vi "OE1022D_Common_Query Data.vi"(0 "VISA resource name":refnum<visa-resource-name>, 1 "OE1022D_Query Multi Data":T2 {"Query Type 5" items=["X", "Y", "R", "θ", "Freq", "Xh1", "Yh1", "Rh1", "θh1", "Xh2", "Yh2", "Rh2", "θh2", "Noise", "A1", "A2", "A3", "A4", "E1", "E2", "E3", "E4"]; "Query Type 4" items=["X", "Y", "R", "θ", "Freq", "Xh1", "Yh1", "Rh1", "θh1", "Xh2", "Yh2", "Rh2", "θh2", "Noise", "A1", "A2", "A3", "A4", "E1", "E2", "E3", "E4"]; "Query Type 3" items=["X", "Y", "R", "θ", "Freq", "Xh1", "Yh1", "Rh1", "θh1", "Xh2", "Yh2", "Rh2", "θh2", "Noise", "A1", "A2", "A3", "A4", "E1", "E2", "E3", "E4"]; "Query Type 2" items=["X", "Y", "R", "θ", "Freq", "Xh1", "Yh1", "Rh1", "θh1", "Xh2", "Yh2", "Rh2", "θh2", "Noise", "A1", "A2", "A3", "A4", "E1", "E2", "E3", "E4"]; "Query Type 1" items=["X", "Y", "R", "θ", "Freq", "Xh1", "Yh1", "Rh1", "θh1", "Xh2", "Yh2", "Rh2", "θh2", "Noise", "A1", "A2", "A3", "A4", "E1", "E2", "E3", "E4"]}, 5 "Channel":u16(ring)=1 items=["A"=1, "B"=2], 7 "Remote Mode":u16(ring) items=["USB", "RS232", "GPIB"], 9 "Timeout":u32=1000, 11 "Error in (no error)":errorcluster caption="error out（no error）") -> (4 "VISA resource  out":refnum<visa-resource-name>, 8 "Parameter Values":T1, 10 "Output String":string, 15 "Error out":errorcluster caption="error out")   [LabVIEW 2011]
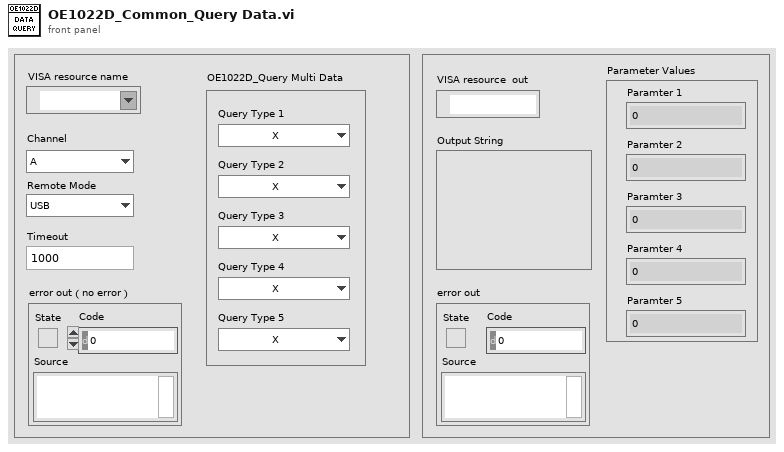
[diagram p1: front panel]
types:
  T1 = cluster{"Paramter 1":dbl, "Paramter 2":dbl, "Paramter 3":dbl, "Paramter 4":dbl, "Paramter 5":dbl}
  T2 = cluster{"Query Type 1":u16, "Query Type 2":u16, "Query Type 3":u16, "Query Type 4":u16, "Query Type 5":u16}
  T3 = enum16{"ISRC", "IGND", "ICPL", "ILIN", "PHAS", "FMOD", "RSLP", "FREQ", "SWPT", "SLLM", "SULM", "SSLL", "SSLG", "STLM", "SWRM", "IRNG", "SENS", "RMOD", "OFLT", "OFSL", "SYNC", "DMOD", "HARM", "DARB", "SWVT", "SLVL", "SVLL", "SVUL", "SVSL", "SVSG", "SVTM", "SVRM", "RALL", "SNAP", "OUTP", "OAUX", "COUT", "CAUX", "COFP", "CEXP", "FPOP", "OEXP", "*IDN", "*RST", "OVLD", "INOV", "GNOV", "*PLL", "SSET", "RSET", "AGAN", "APHS", "ARSV", "ASCL", "EQCD", "EQCS", "SPED", "SRAT", "SLEN", "SSLE", "STRG", "SPRM", "STRD", "PAUS", "REST", "SPTS", "TRCA", "TEMP", "RSTU", "IHNZ", "DEQU", "SADD", "ARNG", "CSPE", "ISRCD", "IGNDD", "ICPLD", "ILIND", "PHASD", "FMODD", "RSLPD", "FREQD", "SWPTD", "SLLMD", "SULMD", "SSLLD", "SSLGD", "STLMD", "SWRMD", "SENSD", "RMODD", "OFLTD", "OFSLD", "SYNCD", "HARMD", "EQCDD", "EQCSD", "SNAPD", "OUTPD", "SWVTD", "SLVLD", "SVLLD", "SVULD", "SVSLD", "SVSGD", "SVTMD", "SVRMD", "SVDCD", "ARSVD", "AGAND", "APHSD", "ASCLD", "FPOPD", "CAUXD", "OEXPD", "SPEDD", "SRATD", "SLEND", "SSLED", "STRGD", "SPRMD", "STRDD", "PAUSD", "RESTD", "SPTSD", "TRCAD", "*IDND", "*RSTD", "INOVD", "GNOVD", "*PLLD", "SSETD", "RSETD", "RALLD"}
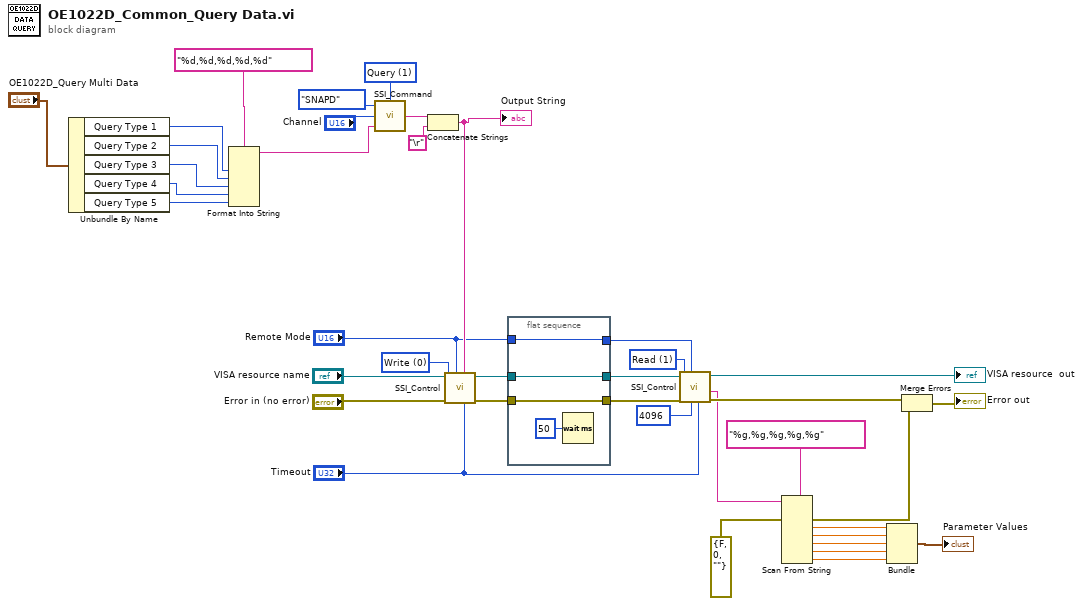
[diagram p0: block diagram]
diagram:
  w27 = u16 1 items=["Set", "Query"] ("Opera")
  w32 = u16 1 items=["Write", "Read"] ("Control")
  w37 = u16 0 items=["Write", "Read"] ("Control")
  n1 = Unbundle By Name("OE1022D_Query Multi Data") -> ("Query Type 1"=w6:u16, "Query Type 2"=w5:u16, "Query Type 3"=w4:u16, "Query Type 4"=w3:u16, "Query Type 5"=w1:u16)
  n2 = Format Into String(format string="%d,%d,%d,%d,%d" ("格式字符串"), w6, w5, w4, w3, w1) -> (resulting string=w7:string)  [unwired: 2 in, 1 out]
  n3 = call "SSI_Command.vi"("Opera"=w27, "Paramter"=w7, "channel"="Channel", "Command Type"=T3."SNAPD") -> ("Output string"=w10:string)
  n4 = Concatenate Strings(w10, "\r") -> (w30:string)
  "Output String" <- w30
  n5 = call "SSI_Control.vi"("Tineout"="Timeout", "Write Buffer"=w30, "Remote Mode"="Remote Mode", "Error in (no error)"="Error in (no error)", "Control"=w37, "VISA resource name"="VISA resource name") -> ("Error out"=w35:errorcluster, "VISA resource  out"=w36:refnum<visa-resource-name>)  [unwired: 2 in, 2 out]
  n6 = flat-sequence {
    tunnel: w36 -> [w43]
    tunnel: w35 -> [w42]
    tunnel: [w43] -> w34
    tunnel: [w42] -> w33
    tunnel: [w40] -> w17
    tunnel: "Remote Mode" -> [w40]
    frame #0 {
      n7 = Wait (ms)(milliseconds to wait=u32 50 ("等待时间（毫秒）")) -> ()  [unwired: 1 out]
    }
  }
  n8 = call "SSI_Control.vi"("Tineout"="Timeout", "Number of bytes"=u32 4096, "Remote Mode"=w17, "Error in (no error)"=w33, "Control"=w32, "VISA resource name"=w34) -> ("Error out"=w16:errorcluster, "Read Buffer"=w14:string, "VISA resource  out"=→"VISA resource  out":refnum<visa-resource-name>)  [unwired: 2 in, 1 out]
  n9 = Scan From String(format string="%g,%g,%g,%g,%g" ("格式字符串"), input string=w14, error in=errorcluster {"status"=FALSE, "code"=0, "source"=""} ("error constant")) -> (error out=w13:errorcluster, output 1=w22:dbl, output 2=w21:dbl, output 3=w23:dbl, output 4=w24:dbl, output 5=w25:dbl)  [unwired: 6 in, 2 out]
  n10 = Bundle(w22, w21, w23, w24, w25) -> (→"Parameter Values":cluster{dbl, dbl, dbl, dbl, dbl})  [unwired: 1 in]
  n11 = Merge Errors(w16, w13) -> (→"Error out":errorcluster)
